vi "Close Splash.vi"(8 "error in (no error)":errorcluster, 11 "Plugin Splash in":refnum<class "Plugin Splash.lvclass">) -> (0 "error out":errorcluster, 3 "Plugin Splash out":refnum<class "Plugin Splash.lvclass">)   [LabVIEW 2020, in "Volatus.lvlib" / "Plugin Splash.lvclass"]
uses:
  Plugin Splash.lvclass
  Plugin Splash.lvclass/Plugin Splash.ctl
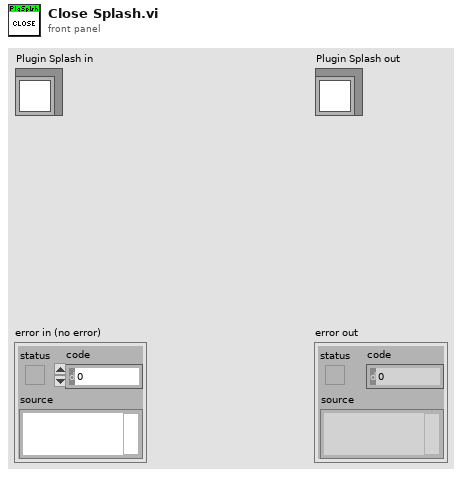
[diagram p1: front panel]
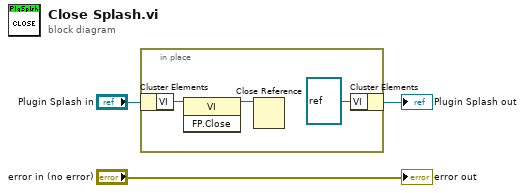
[diagram p0: block diagram]
diagram:
  n1 = in-place {
    n2 = in-place-cluster #1("Plugin Splash in") -> ("VI"=w6:refnum<vi>)
    n3 = invoke class="VI" method="FP.Close"(reference=w6) -> (reference out=w4:refnum<vi>)  [unwired: 2 in, 2 out]
    n4 = Close Reference(reference=w4) -> ()  [unwired: 1 in, 1 out]
    n5 = in-place-cluster #1("VI"=refnum<vi> refnum) -> (→"Plugin Splash out":refnum<class "Plugin Splash.lvclass">)
  }
  "error out" <- "error in (no error)"
